vi "Main Page.vi"(8 "error in (no error)":errorcluster, 11 "Node Ptr":T1 format="%.0x") -> (0 "error out":errorcluster)   [LabVIEW 2013, in "Trigger Timestamp Logging System Explorer.lvlib"]
uses:
  Trigger Timestamp Logging System Explorer.lvlib
  <vilib>/NI Veristand/Custom Device API/Custom Device Item Ref.ctl
  <vilib>/NI Veristand/Custom Device API/Get Item Property (Variant).vi
  <vilib>/NI Veristand/Custom Device API/Set Item Property (Variant).vi
  <vilib>/NI Veristand/Custom Device API/Custom Device API.lvlib
panel:
  in  "XNET Interface Name (Ex: CAN2)":string
  in  "Interface 2 XNET Database":refnum<k21>
  in  "XNET Interface Name (Ex: CAN1)":string
  in  "Interface 1 XNET Database":refnum<k21>
  in  "Header":cluster{"Section Name":string}={"Section Name"="Custom Device Item Settings"}
  in  "Description":string
  in  "Name":string
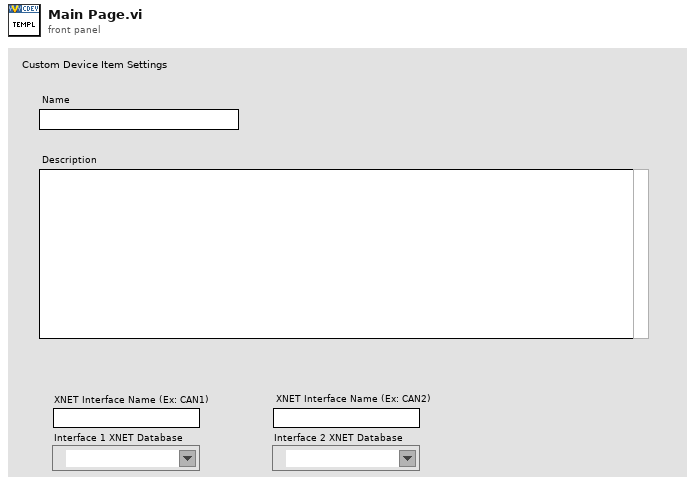
[diagram p1: front panel]
types:
  T1 = typedef "Custom Device API.lvlib/Custom Device Item Ref.ctl" = u64
  T2 = cluster{"Interface1":string, "Interface2":string, "Interface 1 DB":refnum<k21>, "Interface 2 DB":refnum<k21>}
  T3 = typedef "Custom Device API.lvlib/Custom Device Item Info.ctl" = cluster{"Name":string, "Is Channel":bool, "GUID":string, "Is Waveform":bool}
  T4 = typedef "Custom Device API.lvlib/Custom Device Commands.ctl" = enum16{"Default", "Item renamed", "Shutdown", "Dynamic button pressed"}
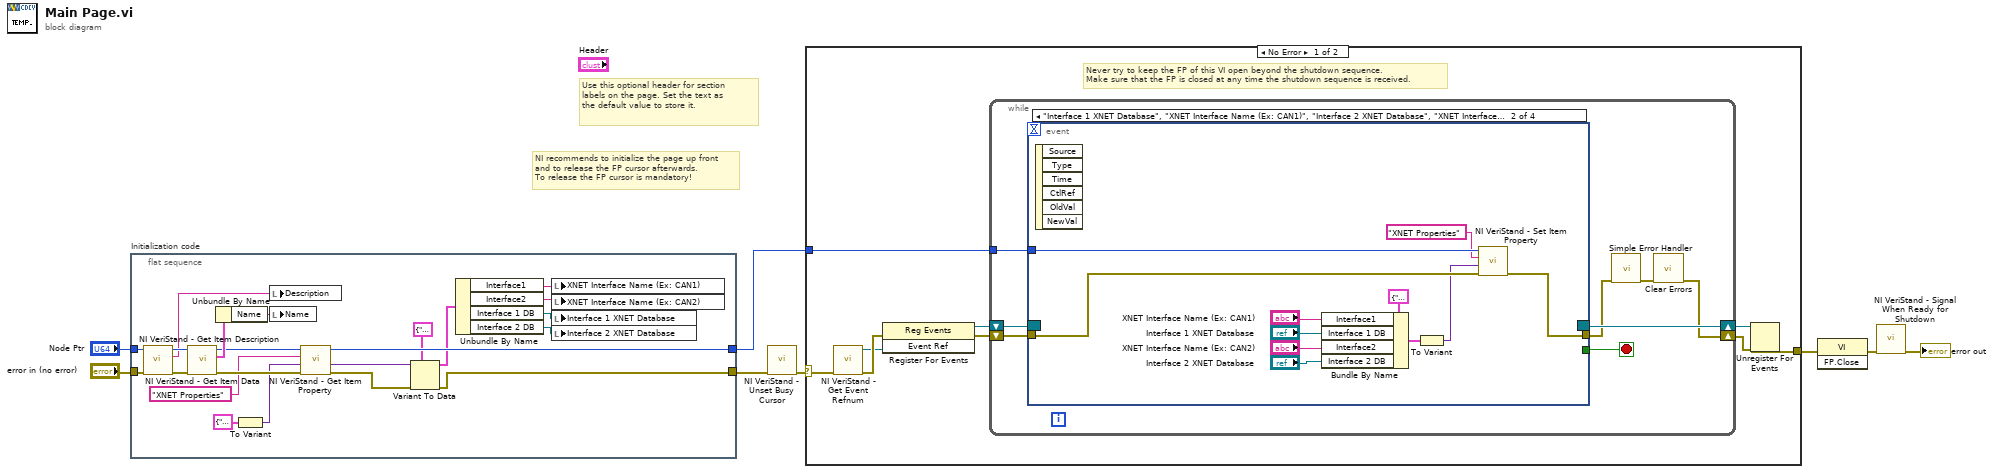
[diagram p0: block diagram]
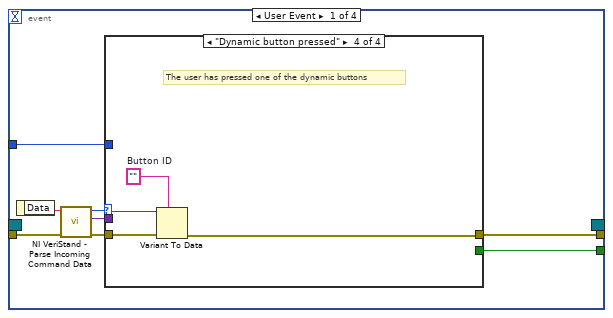
[diagram p2: hidden frame]
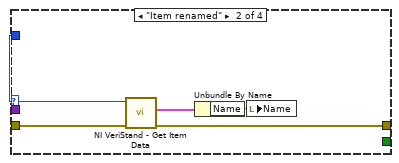
[diagram p4: hidden frame]
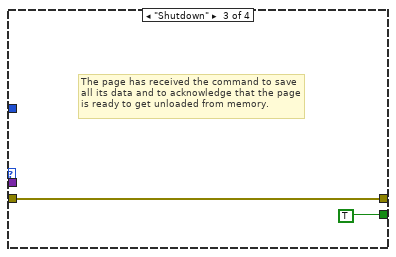
[diagram p5: hidden frame]
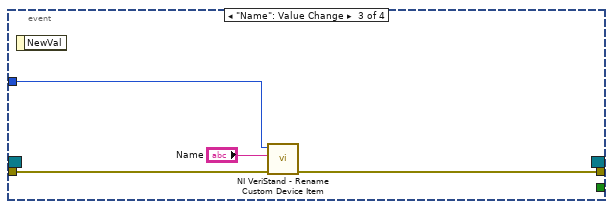
[diagram p6: hidden frame]
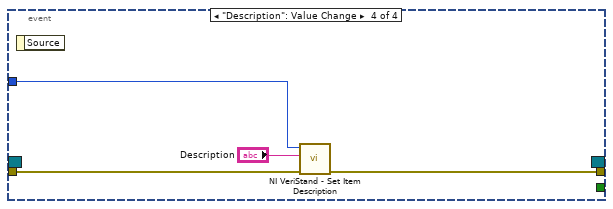
[diagram p7: hidden frame]
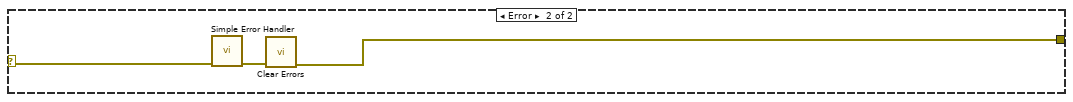
[diagram p8: hidden frame]
diagram:
  # "Use this optional header for section labels on the page. Set the text as the default value to store it."
  # "NI recommends to initialize the page up front\nand to release the FP cursor afterwards.\nTo release the FP cursor is mandatory!"
  n1 = flat-sequence "Initialization code" {
    tunnel: "error in (no error)" -> [w29]
    tunnel: "Node Ptr" -> [w28]
    tunnel: [w14] -> w4
    tunnel: [w18] -> w1
    frame #0 {
      n2 = call <vilib>:"NI VeriStand - Get Item Description.vi"("error in (no error)"=w29, "Item Ref in"=w28) -> ("error out"=w26:errorcluster, "Description"=w27:string, "Item Ref out"=w30:T1)  [unwired: 7 out]
      n3 = call <vilib>:"NI VeriStand - Get Item Data.vi"("error in (no error)"=w26, "Item Ref in"=w30) -> ("error out"=w22:errorcluster, "Item Info"=w25:T3, "Item Ref out"=w23:T1)  [unwired: 7 out]
      n4 = Unbundle By Name(w25) -> ("Name"=w24:string)
      n5 = To Variant(anything=T2 {"Interface1"="", "Interface2"="", "Interface 1 DB"="125kDB", "Interface 2 DB"="125kDB"}) -> (Variant=w19:variant)
      n6 = local write "Description"(w27) -> ()
      n7 = local write "Name"(w24) -> ()
      n8 = call-poly <vilib>:"NI VeriStand - Get Item Property.vi"("error in (no error)"=w22, "Default Value"=w19, "Property Name"="XNET Properties", "Item Ref in"=w23) -> ("error out"=w17:errorcluster, "Value"=w16:variant, "Item Ref out"=w18:T1)  [unwired: 4 in, 1 out]
      n9 = Variant To Data(error in=w17, type=T2 {"Interface1"="", "Interface2"="", "Interface 1 DB"="125kDB", "Interface 2 DB"="125kDB"}, Variant=w16) -> (data=w13:T2, error out=w14:errorcluster)
      n10 = Unbundle By Name(w13) -> ("Interface1"=w12:string, "Interface2"=w11:string, "Interface 1 DB"=w9:refnum<k21>, "Interface 2 DB"=w10:refnum<k21>)
      n11 = local write "XNET Interface Name (Ex: CAN1)"(w12) -> ()
      n12 = local write "XNET Interface Name (Ex: CAN2)"(w11) -> ()
      n13 = local write "Interface 1 XNET Database"(w9) -> ()
      n14 = local write "Interface 2 XNET Database"(w10) -> ()
    }
  }
  n15 = call <vilib>:"NI VeriStand - Unset Busy Cursor.vi"("error in (no error)"=w4) -> ("error out"=w3:errorcluster)  [unwired: 10 out]
  n16 = case shown="No Error" w3 {
    selector: w3 -> [w31 w89]
    tunnel: [w36 w87] -> w8
    tunnel: w1 -> [w32 _]
    frame No Error {
      # "Never try to keep the FP of this VI open beyond the shutdown sequence.\nMake sure that the FP is closed at any time the shutdown sequence is received."
      n17 = call <vilib>:"NI VeriStand - Get Event Refnum.vi"("error in (no error)"=w31) -> ("error out"=w39:errorcluster, "Event Ref"=w35:refnum<user-event>)  [unwired: 9 out]
      n18 = register-events(error in=w39, w35) -> (reference out=w33:refnum<event-registration>, error out=w34:errorcluster)  [unwired: 1 in]
      n19 = while {
        tunnel: w32 -> [w43]
        shift-right: [w40] -> w37
        shift-left: w34 -> [w46]
        shift-right: [w47] -> w38
        shift-left: w33 -> [w45]
        stop <- w44 stop-if-true
        n20 = event shown="[1] \"Interface 1 XNET Database\", \"XNET Interface Name (Ex: CAN1)\", \"Interface 2 XNET Database\", \"XNET Interface Name (Ex: CAN2)\": Value Change" {
          selector: w45 -> [_ _ _ _]
          dyn-events: [_ _ _ _] -> w47
          timeout: _ -> [_ _ _ _]
          tunnel: w46 -> [w55 w71 w82 w85]
          tunnel: [w51 _ _ _] -> w44
          tunnel: [w50 w68 w81 w84] -> w42
          tunnel: w43 -> [w49 w72 w80 w86]
          event User Event {
            n21 = event-data() -> ("Data"=w54:string)  [unwired: 1 out]
            n22 = call <vilib>:"NI VeriStand - Parse Incoming Command Data.vi"("error in (no error)"=w55, "Incoming data"=w54) -> ("error out"=w53:errorcluster, "Outgoing data"=w48:variant, "Action"=w52:T4)  [unwired: 7 out]
            n23 = case shown="\"Dynamic button pressed\"" w52 {
              tunnel: w53 -> [w56 w61 w62 w67]
              tunnel: [_ _ TRUE _] -> w51
              tunnel: [w56 w58 w62 w64] -> w50
              tunnel: w49 -> [_ w60 _ _]
              tunnel: w48 -> [_ _ _ w66]
              frame "Default", Default {
              }
              frame "Item renamed" {
                n24 = call <vilib>:"NI VeriStand - Get Item Data.vi"("error in (no error)"=w61, "Item Ref in"=w60) -> ("error out"=w58:errorcluster, "Item Info"=w59:T3)  [unwired: 8 out]
                n25 = Unbundle By Name(w59) -> ("Name"=w57:string)
                n26 = local write "Name"(w57) -> ()
              }
              frame "Shutdown" {
                # "The page has received the command to save all its data and to acknowledge that the page is ready to get unloaded from memory."
              }
              frame "Dynamic button pressed" {
                w65 = ""  # Button ID
                # "The user has pressed one of the dynamic buttons"
                n27 = Variant To Data(error in=w67, type=w65, Variant=w66) -> (error out=w64:errorcluster)  [unwired: 1 out]
              }
            }
          }
          event "Interface 1 XNET Database", "XNET Interface Name (Ex: CAN1)", "Interface 2 XNET Database", "XNET Interface Name (Ex: CAN2)": Value Change {
            n28 = event-data() -> ()  [unwired: 7 out]
            n29 = Bundle By Name(cluster=T2 {"Interface1"="", "Interface2"="", "Interface 1 DB"="125kDB", "Interface 2 DB"="125kDB"}, "Interface1"="XNET Interface Name (Ex: CAN1)", "Interface 1 DB"="Interface 1 XNET Database", "Interface2"="XNET Interface Name (Ex: CAN2)", "Interface 2 DB"="Interface 2 XNET Database") -> (w73:T2)
            n30 = To Variant(anything=w73) -> (Variant=w70:variant)
            n31 = call-poly <vilib>:"NI VeriStand - Set Item Property.vi"("error in (no error)"=w71, "Value"=w70, "Property Name"="XNET Properties", "Item Ref in"=w72) -> ("error out"=w68:errorcluster)  [unwired: 5 in, 2 out]
          }
          event "Name": Value Change {
            n32 = event-data() -> ()  [unwired: 2 out]
            n33 = call <vilib>:"NI VeriStand - Rename Custom Device Item.vi"("error in (no error)"=w82, "New Name"="Name", "Item Ref in"=w80) -> ("error out"=w81:errorcluster)  [unwired: 1 in, 7 out]
          }
          event "Description": Value Change {
            n34 = event-data() -> ()  [unwired: 2 out]
            n35 = call <vilib>:"NI VeriStand - Set Item Description.vi"("error in (no error)"=w85, "Description"="Description", "Item Ref in"=w86) -> ("error out"=w84:errorcluster)  [unwired: 8 out]
          }
        }
        n36 = call <vilib>:"Simple Error Handler.vi"("error in (no error)"=w42) -> ("error out"=w41:errorcluster)  [unwired: 1 in, 7 out]
        n37 = call <vilib>:"Clear Errors.vi"("error in (no error)"=w41) -> ("error out"=w40:errorcluster)  [unwired: 6 out]
      }
      n38 = Unregister For Events(event registration refnum=w38, error in=w37) -> (error out=w36:errorcluster)
    }
    frame Error {
      n39 = call <vilib>:"Simple Error Handler.vi"("error in (no error)"=w89) -> ("error out"=w88:errorcluster)  [unwired: 1 in, 7 out]
      n40 = call <vilib>:"Clear Errors.vi"("error in (no error)"=w88) -> ("error out"=w87:errorcluster)  [unwired: 6 out]
    }
  }
  n41 = invoke class="VI" method="FP.Close"(error in=w8) -> (error out=w7:errorcluster)  [unwired: 2 in, 2 out]
  n42 = call <vilib>:"NI VeriStand - Signal When Ready for Shutdown.vi"("error in (no error)"=w7) -> ("error out"=→"error out":errorcluster)  [unwired: 10 out]
